vi "FormatODBPath.vi"(10 "VarName":string, 11 "Category":string) -> (3 "ODB variable path":string)   [LabVIEW 2018, in "feGEM DataPacker.lvlib"]
uses:
  feGEM DataPacker.lvlib
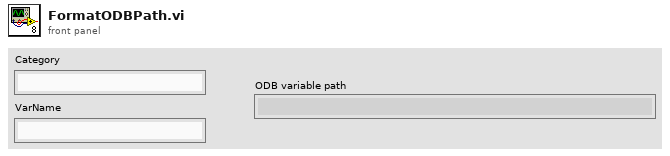
[diagram p1: front panel]
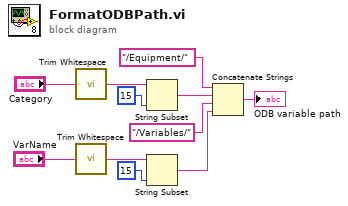
[diagram p0: block diagram]
diagram:
  n1 = call <vilib>:"Trim Whitespace.vi"("string"="Category") -> ("trimmed string"=w10:string)  [unwired: 1 in]
  n2 = call <vilib>:"Trim Whitespace.vi"("string"="VarName") -> ("trimmed string"=w8:string)  [unwired: 1 in]
  n3 = String Subset(string=w10, length (rest)=15 ("length (rest)")) -> (substring=w4:string)  [unwired: 1 in]
  n4 = String Subset(string=w8, length (rest)=15 ("length (rest)")) -> (substring=w2:string)  [unwired: 1 in]
  n5 = Concatenate Strings("/Equipment/" ("string"), w4, "/Variables/" ("string"), w2) -> (→"ODB variable path":string)
